vi "Event Handle Loop.vi"(8 "error in (no error)":errorcluster, 11 "QTab Class in":refnum<class "QTab Class.lvclass">) -> (0 "error out":errorcluster, 3 "QTab Class out":refnum<class "QTab Class.lvclass">)   [LabVIEW 2020, in "QTab.lvlib" / "QTab Class.lvclass"]
uses:
  QTab Class.lvclass
  QTab Class.lvclass/QTab Class.ctl
  Pag Attribute.ctl
panel:
  out "Picture":picture
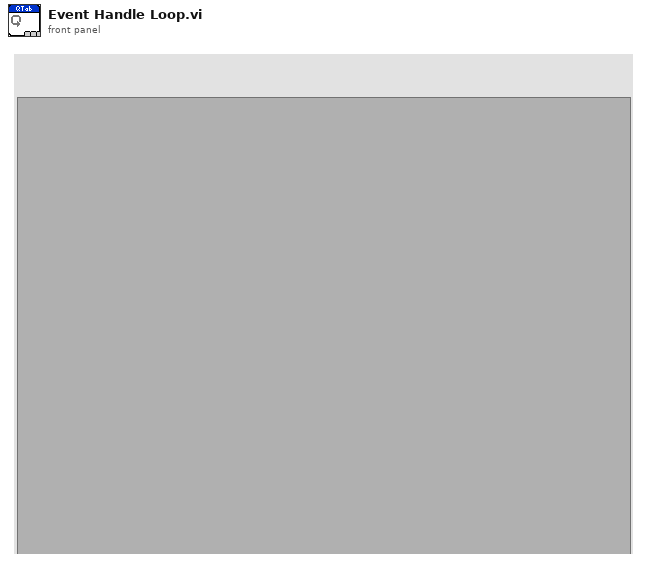
[diagram p1: front panel]
types:
  T1 = typedef "QTab.lvlib/QTab Class.lvclass/Pag Attribute.ctl" = cluster{"VI Refnum":refnum<vi>, "Page Name":string, "Closeable":bool, "Draggable":bool, "Pop-Out":bool}
  T2 = typedef "QTab.lvlib/QTab Class.lvclass/Command.ctl" = enum16{"Startup", "Add Page", "Close All Page", "Set Page Attribute", "Pop-out", "Merage", "Insert", "Stop"}
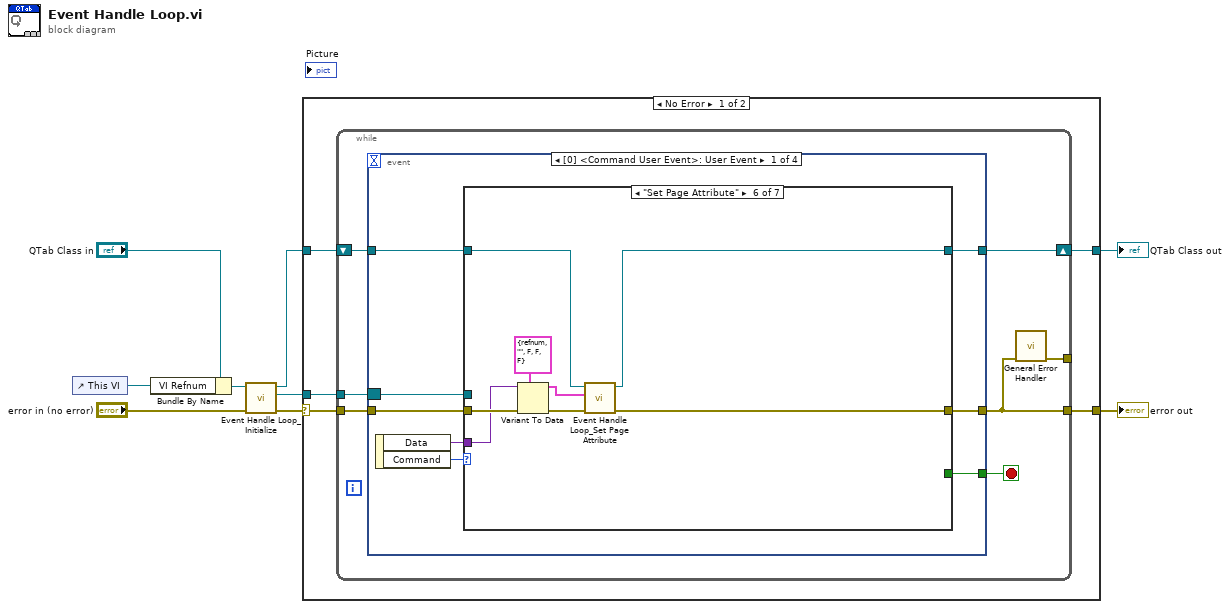
[diagram p0: block diagram]
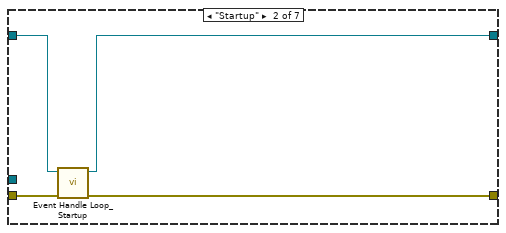
[diagram p3: hidden frame]
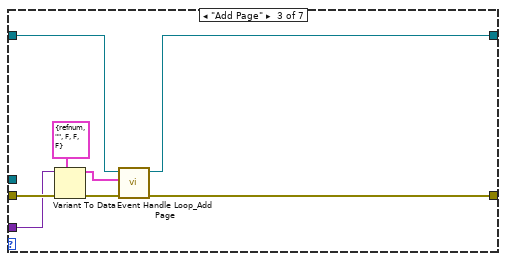
[diagram p4: hidden frame]
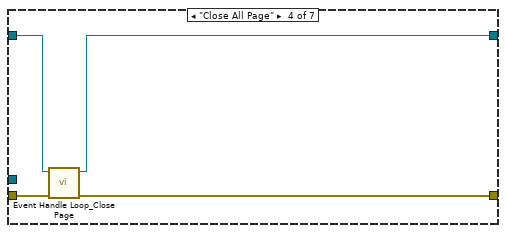
[diagram p5: hidden frame]
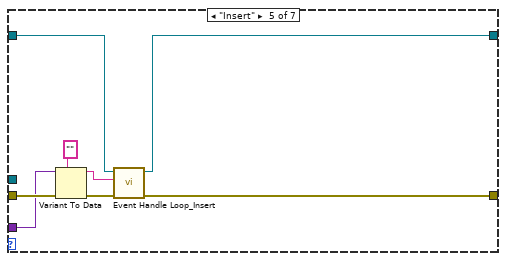
[diagram p6: hidden frame]
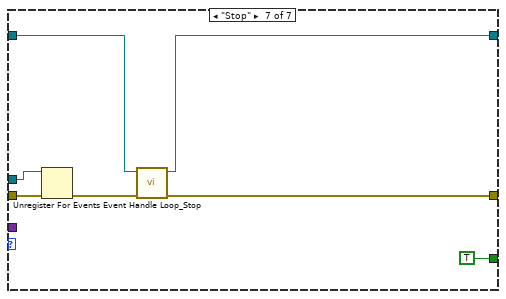
[diagram p7: hidden frame]
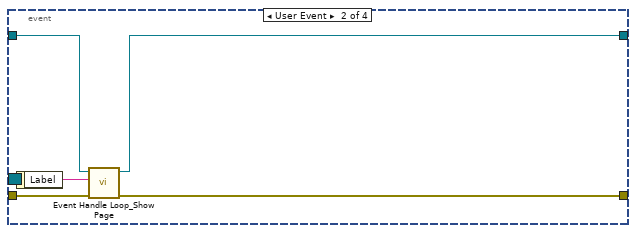
[diagram p8: hidden frame]
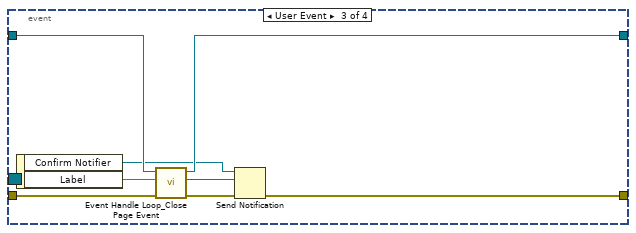
[diagram p9: hidden frame]
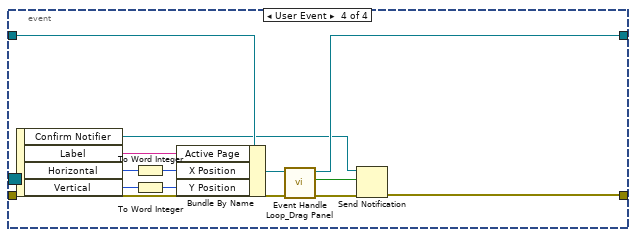
[diagram p10: hidden frame]
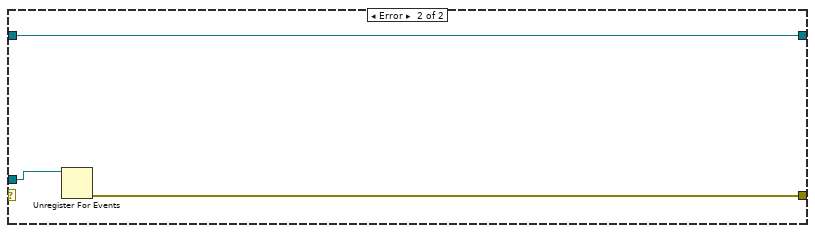
[diagram p11: hidden frame]
diagram:
  n1 = control-ref of="This VI"() -> (w7:refnum<vi>)
  n2 = Bundle By Name(cluster="QTab Class in", "VI Refnum"=w7) -> (w2:refnum<class "QTab Class.lvclass">)
  n3 = call "Event Handle Loop_Initialize.vi"("error in (no error)"="error in (no error)", "QTab Class in"=w2) -> ("error out"=w6:errorcluster, "Event Refnum"=w1:refnum<event-registration>, "QTab Class out"=w5:refnum<class "QTab Class.lvclass">)  [unwired: 7 in]
  n4 = case shown="No Error" w6 {
    selector: w6 -> [w10 _]
    tunnel: w1 -> [w14 w99]
    tunnel: w5 -> [w13 w97]
    tunnel: [w12 w97] -> w9
    tunnel: [w11 w98] -> w8
    frame No Error {
      n5 = while {
        tunnel: w10 -> [w21]
        tunnel: w14 -> [w20]
        tunnel: [w16] -> w11
        shift-right: [w18] -> w12
        shift-left: w13 -> [w19]
        tunnel: [w15] -> _
        stop <- w17 stop-if-true
        n6 = event shown="[0] <Command User Event>: User Event" {
          selector: w20 -> [w26 _ _ _]
          dyn-events: _ -> [_ _ _ _]
          timeout: _ -> [_ _ _ _]
          tunnel: w21 -> [w27 w75 w83 w96]
          tunnel: w19 -> [w25 w73 w82 w94]
          tunnel: [w24 w72 w81 w95] -> w18
          tunnel: [w23 w71 w76 w84] -> w16
          tunnel: [w22 _ _ _] -> w17
          event User Event {
            n7 = event-data() -> ("Data"=w28:variant, "Command"=w29:T2)  [unwired: 1 in]
            n8 = case shown="\"Set Page Attribute\"" w29 {
              tunnel: w28 -> [_ _ w42 _ w54 w62 _]
              tunnel: w27 -> [w30 w35 w43 w44 w55 w63 w70]
              tunnel: w26 -> [_ _ _ _ _ _ w69]
              tunnel: w25 -> [w31 w34 w38 w47 w50 w59 w66]
              tunnel: [w31 w33 w37 w46 w49 w57 w65] -> w24
              tunnel: [w30 w32 w36 w45 w48 w56 w64] -> w23
              tunnel: [_ _ _ _ _ _ TRUE] -> w22
              frame Default {
              }
              frame "Startup" {
                n9 = call "Event Handle Loop_Startup.vi"("error in (no error)"=w35, "QTab Class in"=w34) -> ("error out"=w32:errorcluster, "QTab Class out"=w33:refnum<class "QTab Class.lvclass">)  [unwired: 8 in]
              }
              frame "Add Page" {
                n10 = Variant To Data(error in=w43, type=T1 {"VI Refnum"=refnum, "Page Name"="", "Closeable"=FALSE, "Draggable"=FALSE, "Pop-Out"=FALSE} ("Pag Attribute"), Variant=w42) -> (data=w39:T1, error out=w40:errorcluster)
                n11 = call "Event Handle Loop_Add Page.vi"("error in (no error)"=w40, "Pag Attribute"=w39, "QTab Class in"=w38) -> ("error out"=w36:errorcluster, "QTab Class out"=w37:refnum<class "QTab Class.lvclass">)  [unwired: 7 in]
              }
              frame "Close All Page" {
                n12 = call "Event Handle Loop_Close Page.vi"("error in (no error)"=w44, "QTab Class in"=w47) -> ("error out"=w45:errorcluster, "QTab Class out"=w46:refnum<class "QTab Class.lvclass">)  [unwired: 8 in]
              }
              frame "Insert" {
                n13 = Variant To Data(error in=w55, type="", Variant=w54) -> (data=w51:string, error out=w52:errorcluster)
                n14 = call "Event Handle Loop_Insert.vi"("error in (no error)"=w52, "Label"=w51, "QTab Class in"=w50) -> ("error out"=w48:errorcluster, "QTab Class out"=w49:refnum<class "QTab Class.lvclass">)  [unwired: 7 in]
              }
              frame "Set Page Attribute" {
                n15 = Variant To Data(error in=w63, type=T1 {"VI Refnum"=refnum, "Page Name"="", "Closeable"=FALSE, "Draggable"=FALSE, "Pop-Out"=FALSE} ("Pag Attribute"), Variant=w62) -> (data=w58:T1, error out=w60:errorcluster)
                n16 = call "Event Handle Loop_Set Page Attribute.vi"("error in (no error)"=w60, "Pag Attribute"=w58, "QTab Class in"=w59) -> ("error out"=w56:errorcluster, "QTab Class out"=w57:refnum<class "QTab Class.lvclass">)  [unwired: 7 in]
              }
              frame "Stop" {
                n17 = Unregister For Events(event registration refnum=w69, error in=w70) -> (error out=w67:errorcluster)
                n18 = call "Event Handle Loop_Stop.vi"("error in (no error)"=w67, "QTab Class in"=w66) -> ("error out"=w64:errorcluster, "QTab Class out"=w65:refnum<class "QTab Class.lvclass">)  [unwired: 8 in]
              }
            }
          }
          event User Event {
            n19 = event-data() -> ("Label"=w74:string)  [unwired: 1 in]
            n20 = call "Event Handle Loop_Show Page.vi"("error in (no error)"=w75, "Page ID"=w74, "QTab Class in"=w73) -> ("error out"=w71:errorcluster, "QTab Class out"=w72:refnum<class "QTab Class.lvclass">)  [unwired: 7 in]
          }
          event User Event {
            n21 = event-data() -> ("Confirm Notifier"=w78:refnum<notifier>, "Label"=w80:string)  [unwired: 1 in]
            n22 = call "Event Handle Loop_Close Page Event.vi"("error in (no error)"=w83, "Label"=w80, "QTab Class in"=w82) -> ("error out"=w79:errorcluster, "Confirm"=w77:bool, "QTab Class out"=w81:refnum<class "QTab Class.lvclass">)  [unwired: 6 in]
            n23 = Send Notification(notification=w77, notifier=w78, error in (no error)=w79) -> (error out=w76:errorcluster)  [unwired: 1 out]
          }
          event User Event {
            n24 = event-data() -> ("Confirm Notifier"=w86:refnum<notifier>, "Label"=w92:string, "Horizontal"=w91:i32, "Vertical"=w89:i32)  [unwired: 1 in]
            n25 = To Word Integer(number=w91) -> (16bit integer=w90:i16)
            n26 = To Word Integer(number=w89) -> (16bit integer=w88:i16)
            n27 = Bundle By Name(cluster=w94, "Active Page"=w92, "X Position"=w90, "Y Position"=w88) -> (w93:refnum<class "QTab Class.lvclass">)
            n28 = call "Event Handle Loop_Drag Panel.vi"("error in (no error)"=w96, "QTab Class in"=w93) -> ("error out"=w87:errorcluster, "Confirm"=w85:bool, "QTab Class out"=w95:refnum<class "QTab Class.lvclass">)  [unwired: 7 in]
            n29 = Send Notification(notification=w85, notifier=w86, error in (no error)=w87) -> (error out=w84:errorcluster)  [unwired: 1 out]
          }
        }
        n30 = call <vilib>:"General Error Handler.vi"("error in (no error)"=w16) -> ("error out"=w15:errorcluster)  [unwired: 10 in, 4 out]
      }
    }
    frame Error {
      n31 = Unregister For Events(event registration refnum=w99) -> (error out=w98:errorcluster)  [unwired: 1 in]
    }
  }
  "error out" <- w8
  "QTab Class out" <- w9
